vi "DCMotorSim_New_MOI.vi"(8 "MeasurementStdDev":T1, 9 "jKgMetersSquared":dbl, 10 "Gearing":dbl=1.0, 11 "GearBox":T2 {"Jr_KgM2" format="%13.5p"; "L_H" format="%13.5p"; "Kt_NMPerAmp" format="%13.5p"; "KvINV_RadPerSecPerVolt" format="%13.5p"; "R_Ohms" format="%13.5p"; "FreeSpeed_RadPerSec" format="%13.5p"; "FreeCurrent_Amps" format="%13.5p"; "StallCurrent_Amps" format="%13.5p"; "StallTorque_NM" format="%13.5p"; "nominalVoltage_Volts" format="%13.5p"}) -> (0 "Error":bool, 3 "DCMotorSim":T3 {"GearBox"."Jr_KgM2" format="%13.5p"; "GearBox"."L_H" format="%13.5p"; "GearBox"."Kt_NMPerAmp" format="%13.5p"; "GearBox"."KvINV_RadPerSecPerVolt" format="%13.5p"; "GearBox"."R_Ohms" format="%13.5p"; "GearBox"."FreeSpeed_RadPerSec" format="%13.5p"; "GearBox"."FreeCurrent_Amps" format="%13.5p"; "GearBox"."StallCurrent_Amps" format="%13.5p"; "GearBox"."StallTorque_NM" format="%13.5p"; "GearBox"."nominalVoltage_Volts" format="%13.5p"})   [LabVIEW 2019, in "Trajectory_Library.lvlib"]
doc: "Creates a simulated flywheel mechanism.\n \nInputs:\n - gearbox -- The type of and number of motors in the flywheel gearbox.\n - gearing -- The gearing of the flywheel (numbers greater than 1 represent reductions).\n - jKgMetersSquared -- The moment of inertia of the flywheel. \n - measurementStdDevs -- The standard deviations of the measurements.\n\nOutputs:\n - outFlyWheelSim -- Updated data cluster\n - Error -- If TRUE, an error occured."
uses:
  Trajectory_Library.lvlib
  DCMOTOR_SIM.ctl
  LINEAR_SYSTEM_SIM.ctl
  LINEAR_SYSTEM.ctl
  <vilib>/Analysis/Matrix/Datatypes/RealMatrix.ctl
  DCMOTOR.CTL
  LinearSystem_New.vi
  MatBuilder_Create.vi
  MatrixHelper_Zero.vi
  MatBuilder_Fill.vi
  Matrix_Ident.vi
  MatrixHelper_CoerceSize.vi
  <vilib>/Analysis/7linalg.llb/Create Special Matrix.vi
  <vilib>/Analysis/7linalg.llb/Create Special Real Matrix.vi
  <vilib>/Analysis/Matrix/NI_Matrix.lvlib
panel:
  # "<1, 1>"
  # "<States, 1>"
  # "<Outputs, 1>"
  # "<Inputs, 1>"
  # "<Outputs, 1>"
  # "<States,States>"
  # "<States,Inputs>"
  # "<Outputs,States>"
  # "<Outputs,Inputs>"
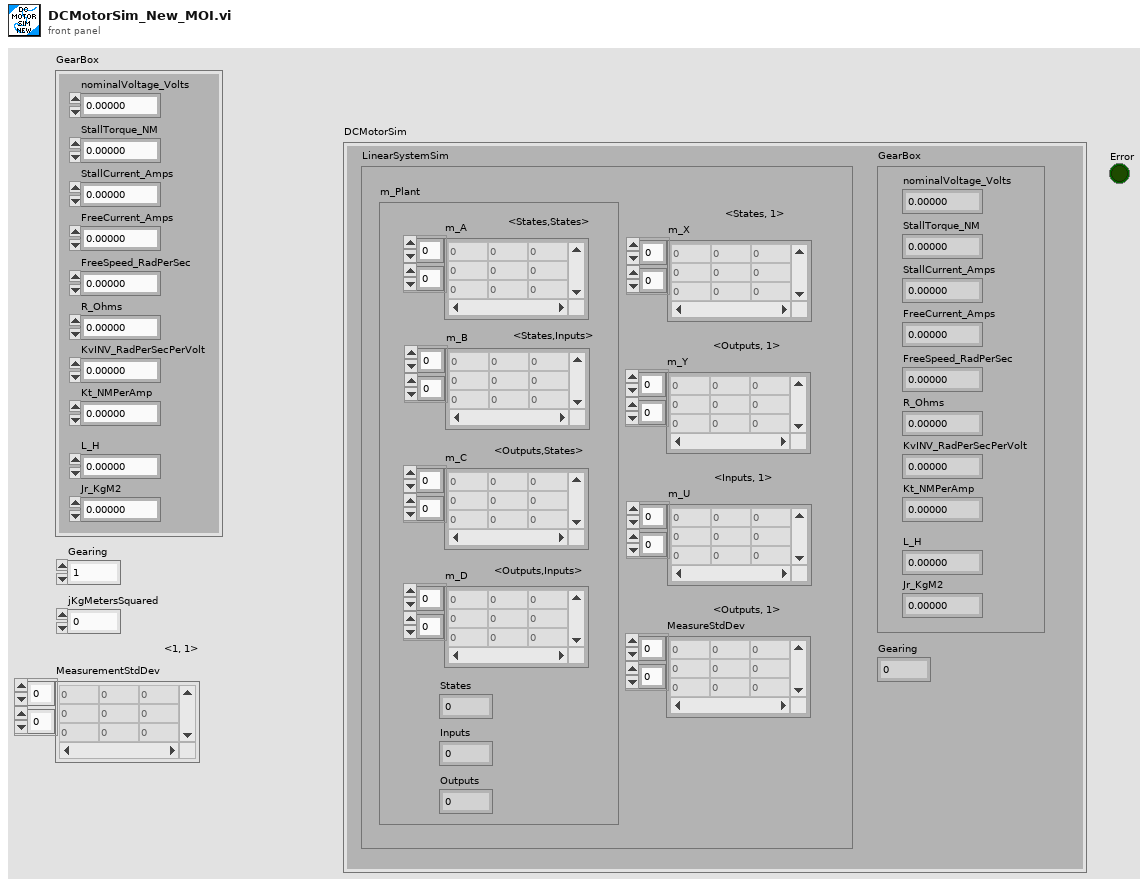
[diagram p1: front panel]
types:
  T1 = typedef "NI_Matrix.lvlib/RealMatrix.ctl" = dbl[][]
  T2 = typedef "Trajectory_Library.lvlib/DCMOTOR.CTL" = cluster{"nominalVoltage_Volts":dbl, "StallTorque_NM":dbl, "StallCurrent_Amps":dbl, "FreeCurrent_Amps":dbl, "FreeSpeed_RadPerSec":dbl, "R_Ohms":dbl, "KvINV_RadPerSecPerVolt":dbl, "Kt_NMPerAmp":dbl, "L_H":dbl, "Jr_KgM2":dbl}
  T3 = typedef "Trajectory_Library.lvlib/DCMOTOR_SIM.ctl" = cluster{"LinearSystemSim":T4, "GearBox":T2, "Gearing":dbl}
  T4 = typedef "Trajectory_Library.lvlib/LINEAR_SYSTEM_SIM.ctl" = cluster{"m_Plant":T5, "m_X":T1, "m_Y":T1, "m_U":T1, "MeasureStdDev":T1}
  T5 = typedef "Trajectory_Library.lvlib/LINEAR_SYSTEM.ctl" = cluster{"m_A":T1, "m_B":T1, "m_C":T1, "m_D":T1, "States":i32, "Inputs":i32, "Outputs":i32}
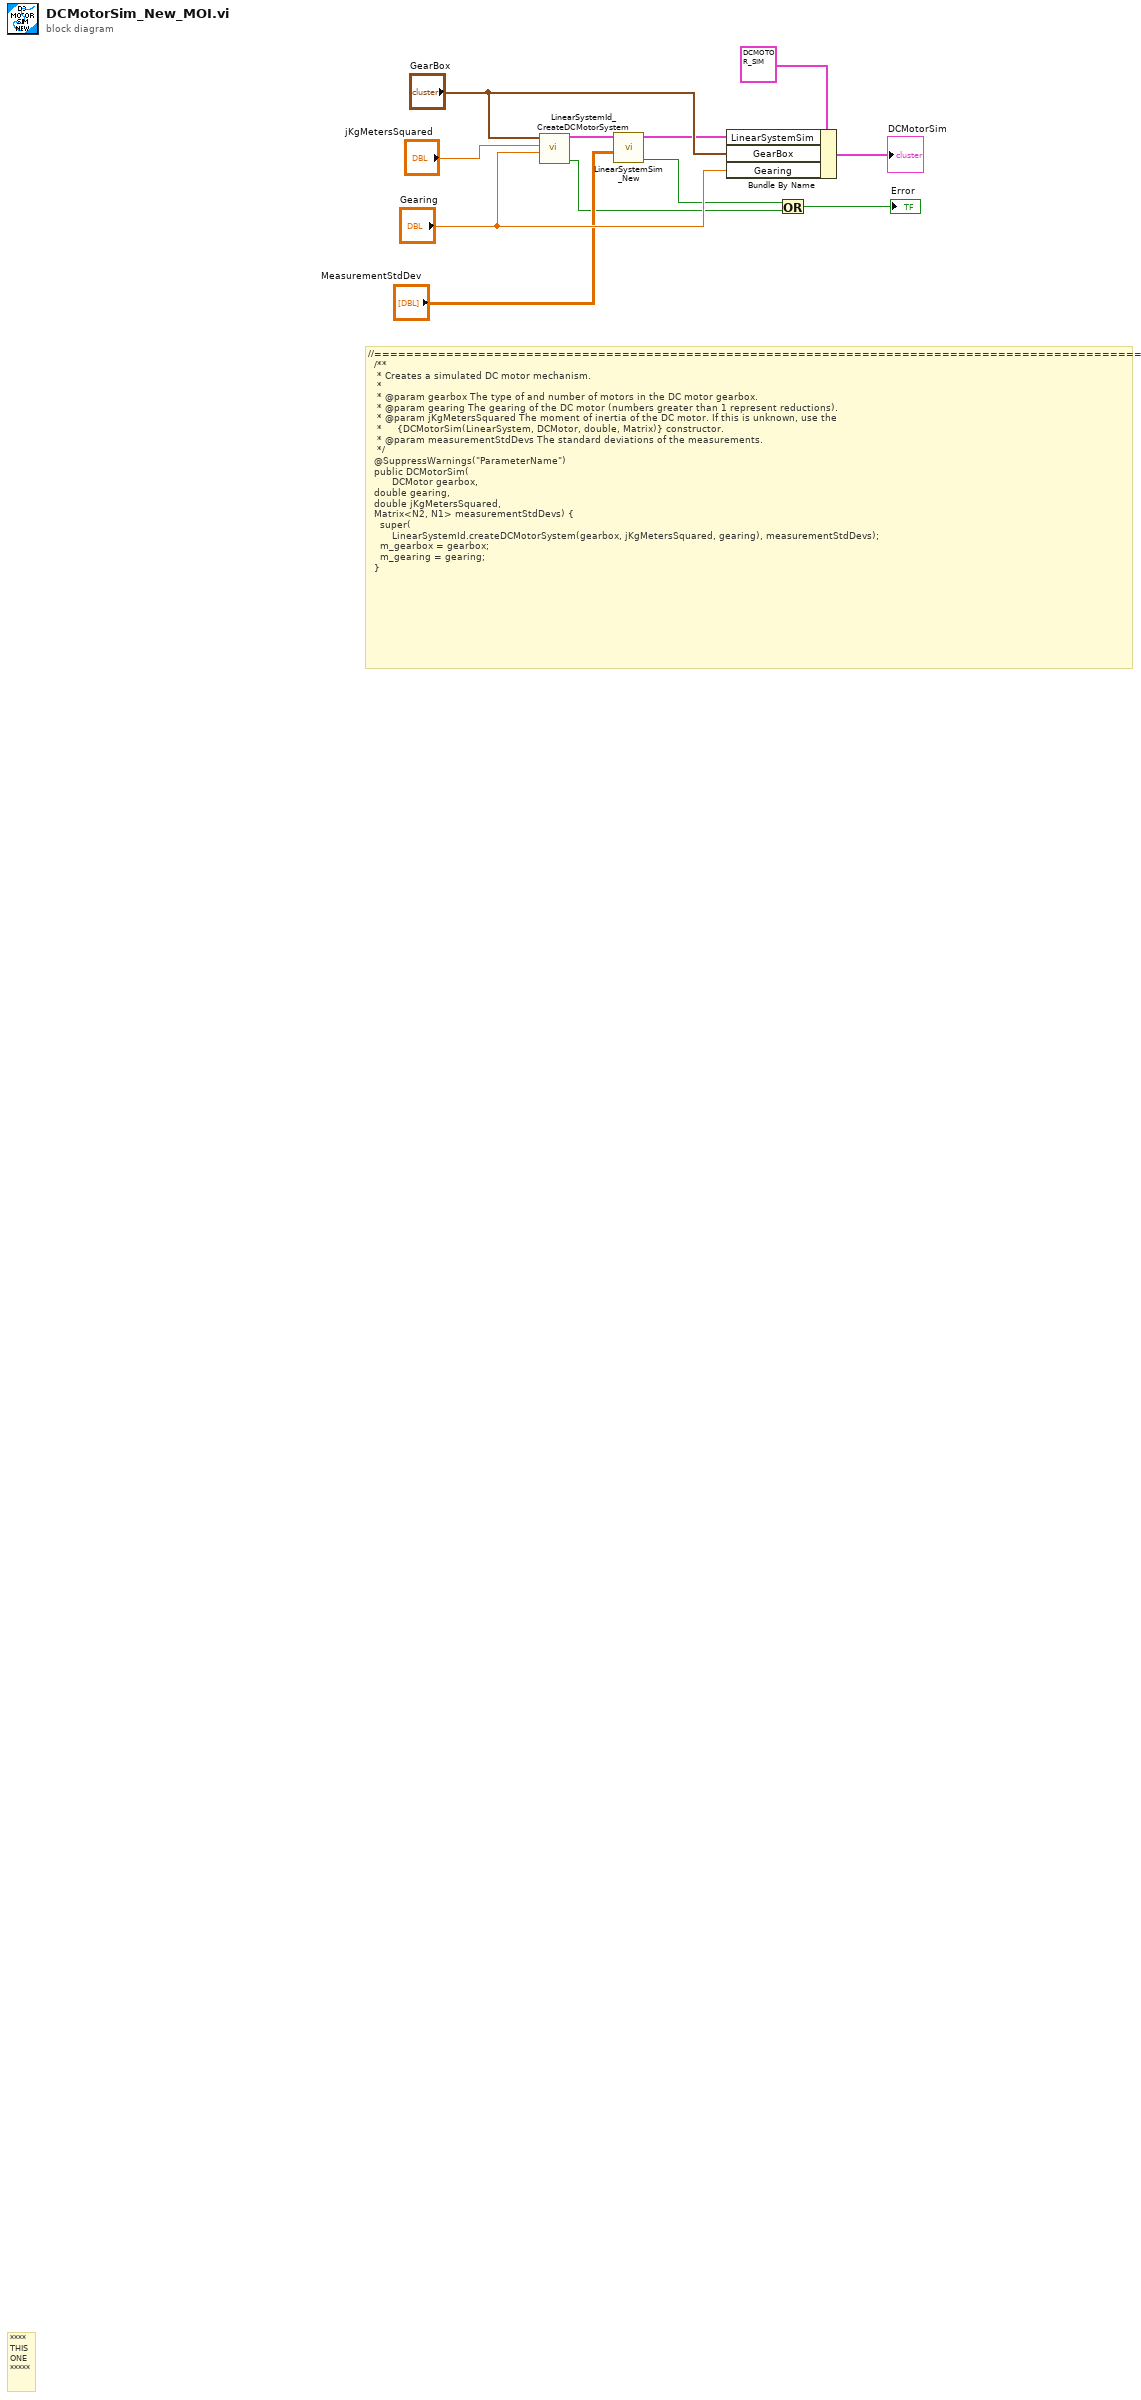
[diagram p0: block diagram]
diagram:
  # "//=================================================================================================\n  /**\n   * Creates a simulated DC motor mechanism.\n   *\n   * @param gearbox The type of and number of motors in the DC motor gearbox.\n   * @param gearing The gearing of the DC motor (numbers greater than 1 represent reductions).\n   * @param jKgMetersSquared The moment of inertia of the DC motor. If this is unknown, use the\n   *     {DCMotorSim(LinearSystem, DCMotor, double, Matrix)} constructor.\n   * @param measurementStdDevs The standard deviations of the measurements.\n   */\n  @SuppressWarnings(\"ParameterName\")\n  public DCMotorSim(\n      \t\tDCMotor gearbox, \n\t\tdouble gearing, \n\t\tdouble jKgMetersSquared, \n\t\tMatrix<N2, N1> measurementStdDevs) {\n    super(\n        LinearSystemId.createDCMotorSystem(gearbox, jKgMetersSquared, gearing), measurementStdDevs);\n    m_gearbox = gearbox;\n    m_gearing = gearing;\n  }"
  # "****\nTHIS\nONE\n*****"
  n1 = call "LinearSystemId_CreateDCMotorSystem.vi"("G"="Gearing", "jKgMetersSquared"="jKgMetersSquared", "DCMOTOR"="GearBox") -> ("Error"=w2:bool, "Linearsystem"=w6:T5)  [unwired: 7 in]
  n2 = call "LinearSystemSim_New.vi"("MeasurementStdDev"="MeasurementStdDev", "System"=w6) -> ("Size Coerced"=w3:bool, "LinearSystemSim"=w4:T4)  [unwired: 8 in]
  n3 = Bundle By Name(cluster=T3 {"LinearSystemSim"={"m_Plant"={"m_A"=[], "m_B"=[], "m_C"=[], "m_D"=[], "States"=0, "Inputs"=0, "Outputs"=0}, "m_X"=[], "m_Y"=[], "m_U"=[], "MeasureStdDev"=[]}, "GearBox"={"nominalVoltage_Volts"=0.0, "StallTorque_NM"=0.0, "StallCurrent_Amps"=0.0, "FreeCurrent_Amps"=0.0, "FreeSpeed_RadPerSec"=0.0, "R_Ohms"=0.0, "KvINV_RadPerSecPerVolt"=0.0, "Kt_NMPerAmp"=0.0, "L_H"=0.0, "Jr_KgM2"=0.0}, "Gearing"=0.0} ("DCMOTOR_SIM"), "LinearSystemSim"=w4, "GearBox"="GearBox", "Gearing"="Gearing") -> (→"DCMotorSim":T3)
  n4 = Or(x=w3, y=w2) -> (x .or. y?=→"Error":bool)
